vi "UI Initialize.vi"(8 "error in (no error)":errorcluster, 11 "UnitTestEngine in":refnum<class "UnitTestEngine.lvclass">) -> (0 "error out":errorcluster, 3 "UnitTestEngine out":refnum<class "UnitTestEngine.lvclass">)   [LabVIEW 2019, in "UnitTestEngine.lvlib" / "UnitTestEngine.lvclass"]
uses:
  UnitTestEngine.lvclass
  C:/Program Files (x86)/National Instruments/LabVIEW 2019/vi.lib/NI/Event Source Actor/Event Source/Event Source/Event Source.lvclass
  TestEngine/TestEngine/TestEngineReference.lvclass
  C:/Program Files (x86)/National Instruments/LabVIEW 2019/vi.lib/NI/Event Source Actor/Event Source/Event/Event.lvclass
  <vilib>/NI/Event Source Actor/Event Source/Event/Event.lvclass/Event.ctl
  UnitTestEngine.lvclass/UnitTestEngine.ctl
  <vilib>/NI/Event Source Actor/Event Source/Event/Event.lvclass
  <vilib>/NI/Event Source Actor/Event Source/Event Source/Event Source.lvclass
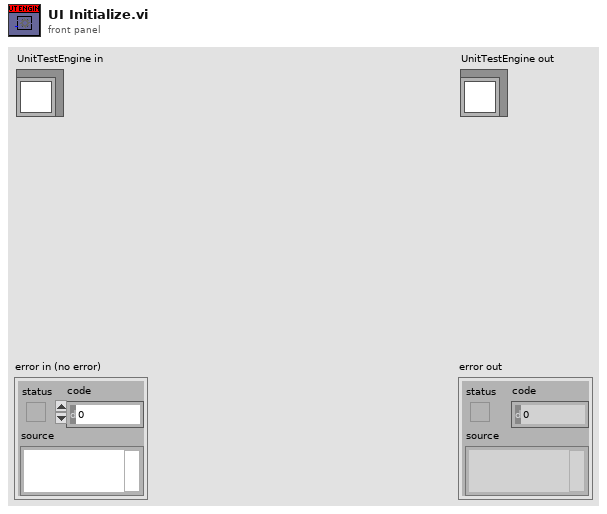
[diagram p1: front panel]
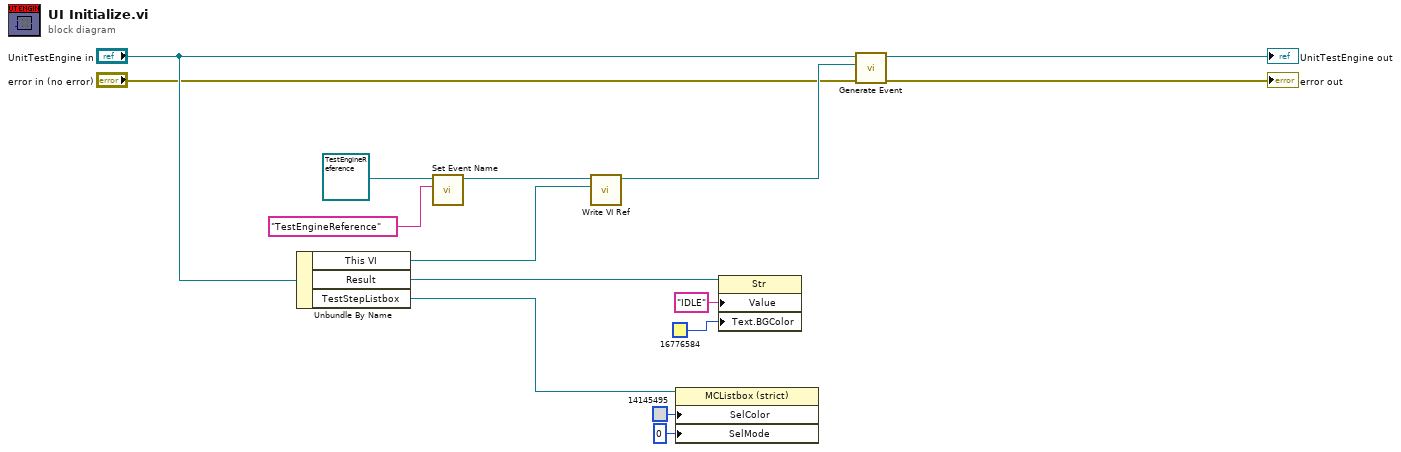
[diagram p0: block diagram]
diagram:
  n1 = Unbundle By Name("UnitTestEngine in") -> ("This VI"=w8:refnum<vi>, "Result"=w11:refnum<vi>, "TestStepListbox"=w3:refnum<vi>)
  n2 = call <vilib>:"Set Event Name.vi"("Name (Generic)"="TestEngineReference", "Event In"=refnum<class "TestEngineReference.lvclass"> refnum ("TestEngine.lvlib:TestEngineReference.lvclass")) -> ("Event Out"=w13:refnum<class "TestEngineReference.lvclass">)  [unwired: 9 in]
  n3 = call-dynamic "Write VI Ref.vi"("VI Ref"=w8, "TestEngineReference in"=w13) -> ("TestEngineReference out"=w12:refnum<class "TestEngineReference.lvclass">)  [unwired: 8 in, 1 out]
  n4 = property class="MCListbox (strict)"(reference=w3, "SelColor"=u32 14145495 ("Selection Color"), "SelMode"=0 ("Selection Mode")) -> ()  [unwired: 1 in, 2 out]
  n5 = property class="Str"(reference=w11, "Value"="IDLE", "Text.BGColor"=u32 16776584 ("Text.Text Colors:BG Color")) -> ()  [unwired: 1 in, 2 out]
  n6 = call <vilib>:"Generate Event.vi"("Error In"="error in (no error)", "Event"=w12, "Event Source In"="UnitTestEngine in") -> ("Error Out"=→"error out":errorcluster, "Event Source Out"=→"UnitTestEngine out":refnum<class "UnitTestEngine.lvclass">)  [unwired: 7 in]
